vi "CPU Info.Set Caches.vi"(8 "error in (no error)":errorcluster, 10 "Caches":T1(array[cluster]), 11 "CPU Info in":refnum<class "CPU Info.lvclass">) -> (0 "error out":errorcluster, 3 "CPU Info out":refnum<class "CPU Info.lvclass">)   [LabVIEW 2017, in "DSF.Engine.lvlib" / "CPU Info.lvclass"]
uses:
  CPU Info.lvclass
  CPU Info.lvclass/CPU Info.ctl
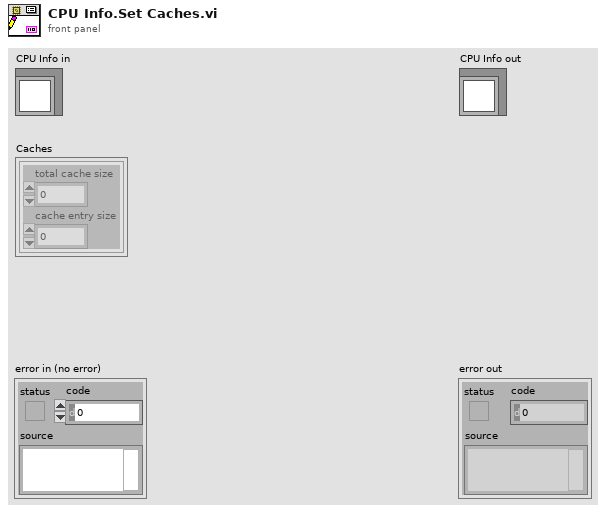
[diagram p1: front panel]
types:
  T1 = cluster{"total cache size":i32, "cache entry size":i32}[]
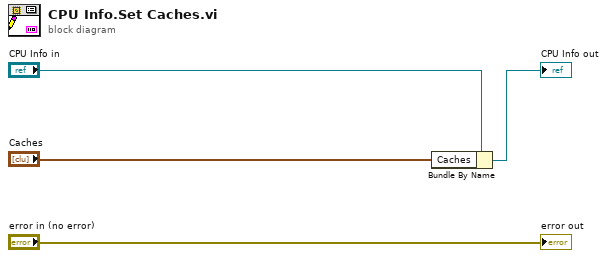
[diagram p0: block diagram]
diagram:
  n1 = Bundle By Name(cluster="CPU Info in", "Caches"="Caches") -> (→"CPU Info out":refnum<class "CPU Info.lvclass">)
  "error out" <- "error in (no error)"
